vi "test_myRio_reloadPrevSettings.vi"(8 "input_error":errorcluster) -> (0 "output_error":errorcluster)   [LabVIEW 2014]
panel:
  out "dataMTrig":bool
  out "dataLC":bool
  out "dataExp":bool
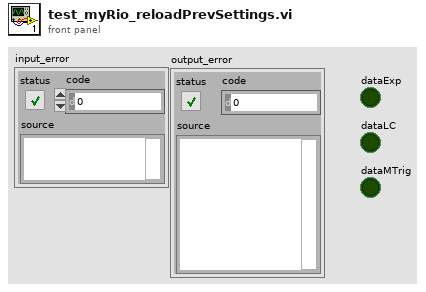
[diagram p1: front panel]
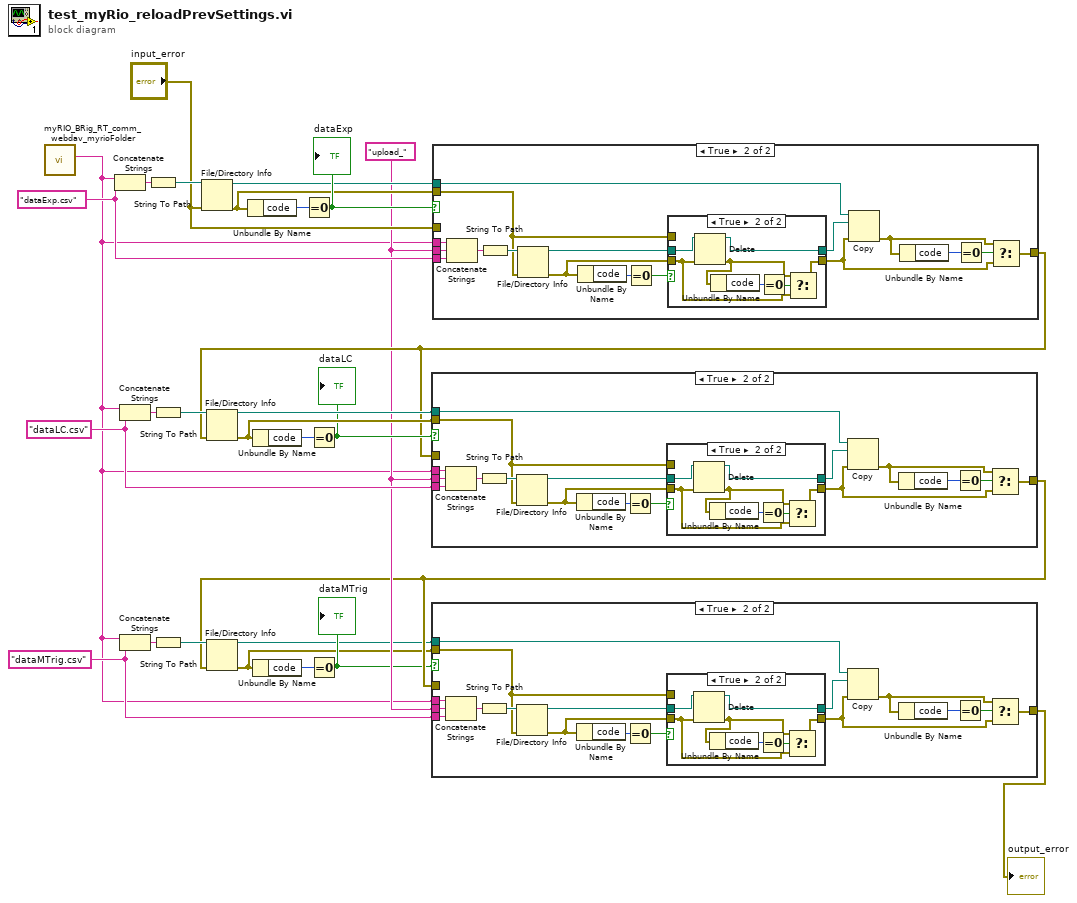
[diagram p0: block diagram]
diagram:
  w8 = "dataMTrig.csv" ("string")
  w10 = "dataLC.csv" ("string")
  w7 = "upload_" ("string")
  w24 = "dataExp.csv" ("string")
  n1 = call "myRIO_BRig_RT_comm_webdav_myrioFolder.vi"() -> ("output_myrioFolder"=w6:string)  [unwired: 11 in]
  n2 = Concatenate Strings(w6, w24) -> (w27:string)
  n3 = Concatenate Strings(w6, w10) -> (w19:string)
  n4 = Concatenate Strings(w6, w8) -> (w16:string)
  n5 = String To Path(string=w27) -> (path=w25:path)
  n6 = String To Path(string=w19) -> (path=w17:path)
  n7 = String To Path(string=w16) -> (path=w14:path)
  n8 = File/Directory Info(path=w25, error in="input_error") -> (path out=w22:path, error out=w21:errorcluster)  [unwired: 5 out]
  n9 = Unbundle By Name(w21) -> ("code"=w26:i32)
  n10 = Equal To 0?(x=w26) -> (x = 0?=w23:bool)
  "dataExp" <- w23
  n11 = case shown="True" w23 {
    tunnel: w6 -> [_ w45]
    tunnel: w24 -> [_ w44]
    tunnel: w7 -> [_ w43]
    tunnel: w22 -> [_ w36]
    tunnel: [w28 w32] -> w9
    tunnel: w21 -> [_ w30]
    tunnel: "input_error" -> [w28 _]
    frame False {
    }
    frame True {
      n12 = Concatenate Strings(w45, w43, w44) -> (w42:string)
      n13 = String To Path(string=w42) -> (path=w41:path)
      n14 = File/Directory Info(path=w41, error in=w30) -> (path out=w38:path, error out=w37:errorcluster)  [unwired: 5 out]
      n15 = Unbundle By Name(w37) -> ("code"=w40:i32)
      n16 = Equal To 0?(x=w40) -> (x = 0?=w39:bool)
      n17 = case shown="True" w39 {
        tunnel: w37 -> [_ w48]
        tunnel: w38 -> [w47 w54]
        tunnel: [w47 w53] -> w35
        tunnel: [w46 w49] -> w29
        tunnel: w30 -> [w46 _]
        frame False {
        }
        frame True {
          n18 = Delete(path (use dialog)=w54, error in=w48) -> (deleted path=w53:path, error out=w51:errorcluster)  [unwired: 3 in, 1 out]
          n19 = Unbundle By Name(w51) -> ("code"=w52:i32)
          n20 = Equal To 0?(x=w52) -> (x = 0?=w50:bool)
          n21 = Select(t=w51, s=w50, f=w48) -> (s? t:f=w49:errorcluster)
        }
      }
      n22 = Copy(8:w29, 10:w35, 11:w36) -> (0:w31:errorcluster)  [unwired: 2 in, 2 out]
      n23 = Unbundle By Name(w31) -> ("code"=w34:i32)
      n24 = Equal To 0?(x=w34) -> (x = 0?=w33:bool)
      n25 = Select(t=w31, s=w33, f=w29) -> (s? t:f=w32:errorcluster)
    }
  }
  n26 = File/Directory Info(path=w17, error in=w9) -> (path out=w13:path, error out=w12:errorcluster)  [unwired: 5 out]
  n27 = Unbundle By Name(w12) -> ("code"=w18:i32)
  n28 = Equal To 0?(x=w18) -> (x = 0?=w11:bool)
  "dataLC" <- w11
  n29 = case shown="True" w11 {
    tunnel: w6 -> [_ w72]
    tunnel: w10 -> [_ w71]
    tunnel: w7 -> [_ w70]
    tunnel: w13 -> [_ w63]
    tunnel: [w55 w59] -> w5
    tunnel: w12 -> [_ w57]
    tunnel: w9 -> [w55 _]
    frame False {
    }
    frame True {
      n30 = Concatenate Strings(w72, w70, w71) -> (w69:string)
      n31 = String To Path(string=w69) -> (path=w68:path)
      n32 = File/Directory Info(path=w68, error in=w57) -> (path out=w65:path, error out=w64:errorcluster)  [unwired: 5 out]
      n33 = Unbundle By Name(w64) -> ("code"=w67:i32)
      n34 = Equal To 0?(x=w67) -> (x = 0?=w66:bool)
      n35 = case shown="True" w66 {
        tunnel: w64 -> [_ w75]
        tunnel: w65 -> [w74 w81]
        tunnel: [w74 w80] -> w62
        tunnel: [w73 w76] -> w56
        tunnel: w57 -> [w73 _]
        frame False {
        }
        frame True {
          n36 = Delete(path (use dialog)=w81, error in=w75) -> (deleted path=w80:path, error out=w78:errorcluster)  [unwired: 3 in, 1 out]
          n37 = Unbundle By Name(w78) -> ("code"=w79:i32)
          n38 = Equal To 0?(x=w79) -> (x = 0?=w77:bool)
          n39 = Select(t=w78, s=w77, f=w75) -> (s? t:f=w76:errorcluster)
        }
      }
      n40 = Copy(8:w56, 10:w62, 11:w63) -> (0:w58:errorcluster)  [unwired: 2 in, 2 out]
      n41 = Unbundle By Name(w58) -> ("code"=w61:i32)
      n42 = Equal To 0?(x=w61) -> (x = 0?=w60:bool)
      n43 = Select(t=w58, s=w60, f=w56) -> (s? t:f=w59:errorcluster)
    }
  }
  n44 = File/Directory Info(path=w14, error in=w5) -> (path out=w2:path, error out=w3:errorcluster)  [unwired: 5 out]
  n45 = Unbundle By Name(w3) -> ("code"=w15:i32)
  n46 = Equal To 0?(x=w15) -> (x = 0?=w4:bool)
  "dataMTrig" <- w4
  n47 = case shown="True" w4 {
    tunnel: w6 -> [_ w99]
    tunnel: w8 -> [_ w98]
    tunnel: w7 -> [_ w97]
    tunnel: w2 -> [_ w90]
    tunnel: [w82 w86] -> w1
    tunnel: w3 -> [_ w84]
    tunnel: w5 -> [w82 _]
    frame False {
    }
    frame True {
      n48 = Concatenate Strings(w99, w97, w98) -> (w96:string)
      n49 = String To Path(string=w96) -> (path=w95:path)
      n50 = File/Directory Info(path=w95, error in=w84) -> (path out=w92:path, error out=w91:errorcluster)  [unwired: 5 out]
      n51 = Unbundle By Name(w91) -> ("code"=w94:i32)
      n52 = Equal To 0?(x=w94) -> (x = 0?=w93:bool)
      n53 = case shown="True" w93 {
        tunnel: w91 -> [_ w102]
        tunnel: w92 -> [w101 w108]
        tunnel: [w101 w107] -> w89
        tunnel: [w100 w103] -> w83
        tunnel: w84 -> [w100 _]
        frame False {
        }
        frame True {
          n54 = Delete(path (use dialog)=w108, error in=w102) -> (deleted path=w107:path, error out=w105:errorcluster)  [unwired: 3 in, 1 out]
          n55 = Unbundle By Name(w105) -> ("code"=w106:i32)
          n56 = Equal To 0?(x=w106) -> (x = 0?=w104:bool)
          n57 = Select(t=w105, s=w104, f=w102) -> (s? t:f=w103:errorcluster)
        }
      }
      n58 = Copy(8:w83, 10:w89, 11:w90) -> (0:w85:errorcluster)  [unwired: 2 in, 2 out]
      n59 = Unbundle By Name(w85) -> ("code"=w88:i32)
      n60 = Equal To 0?(x=w88) -> (x = 0?=w87:bool)
      n61 = Select(t=w85, s=w87, f=w83) -> (s? t:f=w86:errorcluster)
    }
  }
  "output_error" <- w1
